vi "FT10_FPGA_7854R Tester 3.vi"() -> ()   [LabVIEW 2024]
uses:
  <vilib>/FPGAPlugInAG/PXI-7854R/niLvFpga_Open_PXI-7854R.vi
  <vilib>/rvi/interface/common/dynamic/niFpgaDynamicAddResources.vi
  <vilib>/Utility/error.llb/Error Cluster From Error Code.vi
  <vilib>/rvi/errors/niLvFpgaAdjustHostInterfaceError.vi
  <vilib>/FPGAPlugInAG/Dynamic/niLvFpga_Close_Dynamic.vi
  <vilib>/rvi/interface/nirviOpenFPGA/nirviOpenFPGA.xnode
  FPGA Bitfiles/11_12_2024_FT10_FPGA_7854R_Main_Rev3 BitFile.lvbitx
  <vilib>/rvi/interface/nirviReadWriteControl/nirviReadWriteControl.xnode
  <vilib>/rvi/interface/nirviCloseFPGA/nirviCloseFPGA.xnode
  NiFpgaLv.dll
  <vilib>/rvi/interface/Simulation/niFpgaSimulationCallBeginRW.vi
panel:
  in  "Conn1/DIO_0_7 In":bool[](array[boolean])=[FALSE, FALSE, FALSE, FALSE, FALSE, FALSE, FALSE, FALSE]
  in  "Conn1/DIO_8_15 In":bool[](array[boolean])=[FALSE, FALSE, FALSE, FALSE, FALSE, FALSE, FALSE, FALSE]
  out "Conn1/DIO_0_7 Out":bool[](array[boolean])
  out "Conn1/DIO_8_15 Out":bool[](array[boolean])
  out "Conn1/DIO_16_23 Out":bool[](array[boolean])
  in  "Conn1/DIO_16_23 In":bool[](array[boolean])=[FALSE, FALSE, FALSE, FALSE, FALSE, FALSE, FALSE, FALSE]
  out "error out":errorcluster
  in  "error in":errorcluster
  in  "stop":bool
  in  "uSec On":u16=7
  in  "uSec Off":u16=6
  in  "75kHz":bool=TRUE
  in  "Conn2/DIO_0_7 In":bool[](array[boolean])=[FALSE, FALSE, FALSE, FALSE, FALSE, FALSE, FALSE, FALSE]
  in  "Conn2/DIO_8_15 In":bool[](array[boolean])=[FALSE, FALSE, FALSE, FALSE, FALSE, FALSE, FALSE, FALSE]
  out "Conn2/DIO_0_7 Out":bool[](array[boolean])
  out "Conn2/DIO_8_15 Out":bool[](array[boolean])
  out "error out 2":errorcluster
  out "Conn2/DIO_16_23 Out":bool[](array[boolean])
  in  "Conn2/DIO_16_23 In":bool[](array[boolean])=[FALSE, FALSE, FALSE, FALSE, FALSE, FALSE, FALSE, FALSE]
  # "Inputs - Connector 2"
  # "Outputs - Connector 2"
  # "Inputs - Connector 1"
  # "Outputs - Connector 1"
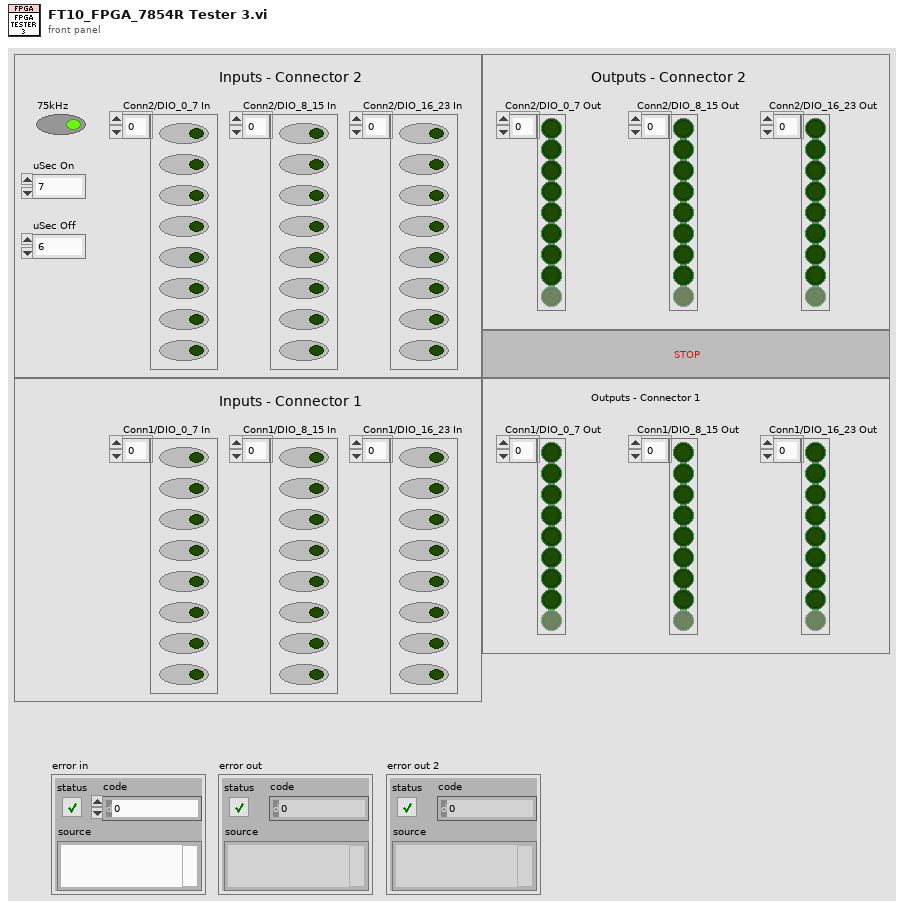
[diagram p1: front panel]
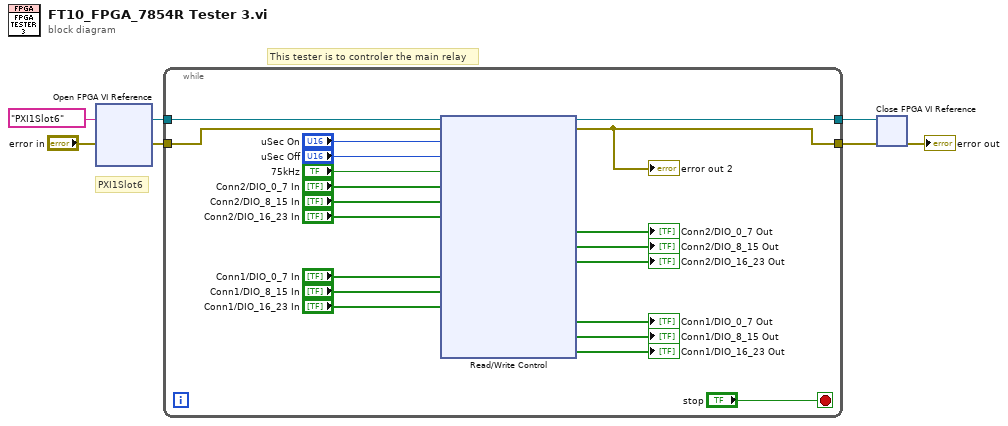
[diagram p0: block diagram]
diagram:
  # "PXI1Slot6"
  # "This tester is to controler the main relay"
  n1 = xnode "Open FPGA VI Reference"("error in"="error in", "resource name"=tag "PXI1Slot6") -> ("FPGA VI Reference Out"=w5:refnum<k20>, "error out"=w4:errorcluster)
  n2 = while {
    tunnel: w5 -> [w27]
    tunnel: [w26] -> w3
    tunnel: w4 -> [w25]
    tunnel: [w24] -> w2
    stop <- "stop" stop-if-true
    n3 = xnode "Read/Write Control"("FPGA VI Reference In"=w27, "error in"=w25, "uSec On"="uSec On", "uSec Off"="uSec Off", "75kHz"="75kHz", "Conn2/DIO_0_7 In"="Conn2/DIO_0_7 In", "Conn2/DIO_8_15 In"="Conn2/DIO_8_15 In", "Conn2/DIO_16_23 In"="Conn2/DIO_16_23 In", "Conn1/DIO_0_7 In"="Conn1/DIO_0_7 In", "Conn1/DIO_8_15 In"="Conn1/DIO_8_15 In", "Conn1/DIO_16_23 In"="Conn1/DIO_16_23 In") -> ("FPGA VI Reference Out"=w26:refnum<k20>, "error out"=w24:errorcluster, "Conn2/DIO_0_7 Out"=→"Conn2/DIO_0_7 Out":bool[], "Conn2/DIO_8_15 Out"=→"Conn2/DIO_8_15 Out":bool[], "Conn2/DIO_16_23 Out"=→"Conn2/DIO_16_23 Out":bool[], "Conn1/DIO_0_7 Out"=→"Conn1/DIO_0_7 Out":bool[], "Conn1/DIO_8_15 Out"=→"Conn1/DIO_8_15 Out":bool[], "Conn1/DIO_16_23 Out"=→"Conn1/DIO_16_23 Out":bool[])
    "error out 2" <- w24
  }
  n4 = xnode "Close FPGA VI Reference"("FPGA VI Reference In"=w3, "error in"=w2) -> ("error out"=→"error out":errorcluster)
